vi "GetDataForExcel.ExtractData.vi"(7 "Report Type":i32, 8 "Error In":errorcluster, 10 "Folders":string[](array[string]), 11 "Path":path) -> (0 "Error Out":errorcluster, 2 "Data":dbl[][](array[numeric]), 3 "Names":string[](array[string]))   [LabVIEW 2013, in "main.lvlib"]
uses:
  main.lvlib
  Controls/Enum Variables.ctl
  <userlib>/_MGI/Error Handling/MGI Suppress Error Code/MGI Suppress Error Code (Scalar).vi
  <userlib>/_OpenG.lib/file/file.llb/File Exists - Scalar__ogtk.vi
  <vilib>/Utility/file.llb/Read From Spreadsheet File (string).vi
  <vilib>/Utility/file.llb/Read From Spreadsheet File (DBL).vi
  <vilib>/regexp/Match Regular Expression.xnode
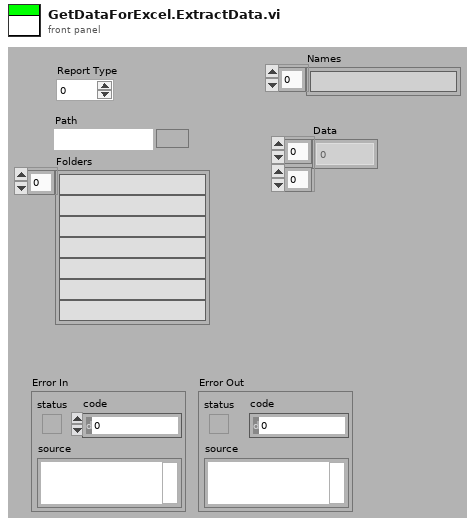
[diagram p1: front panel]
types:
  T1 = typedef "main.lvlib/Enum Variables.ctl" = enum16{"SetAcqFilter", "GetAcqFilter", "Set Filter", "Get Filter", "Set Height", "Get Height", "Set Recorded Height", "Get Recorded Height", "Set Blue Pressure", "Get Blue Pressure", "Set Red Pressure", "Get Red Pressure", "Init", "Reset Pressure", "Set Red Cursors", "Get Red Cursors", "Set Blue Cursors", "Get Blue Cursors", "Set Language", "Get Language", "Set Active Graphs", "Get ActiveGraphs", "Set Method", "Get Method", "Set Encryption", "Get Encryption", "Set ExcelVersion", "Get ExcelVersion", "Set DICOM Avail", "Get DICOM Avail", "Set DICOM Encode", "Get DICOM Encode", "Set JournalExport", "Get JournalExport", "Set Sequence", "Get Sequence", "Set DAQ Connected", "Get DAQ Connected", "Set Current Graph", "Get Current Graph", "Set General Settings", "Get Hyphenation", "Set Arm Calc Method", "Get Arm Calc Method", "Set Dicom Tags", "Get Dicom Tags", "Set BT Serial", "Get BT Serial", "Set BT Accepted Serials", "Get BT Accepted Serials", "Get BT License", "Set BT License"}
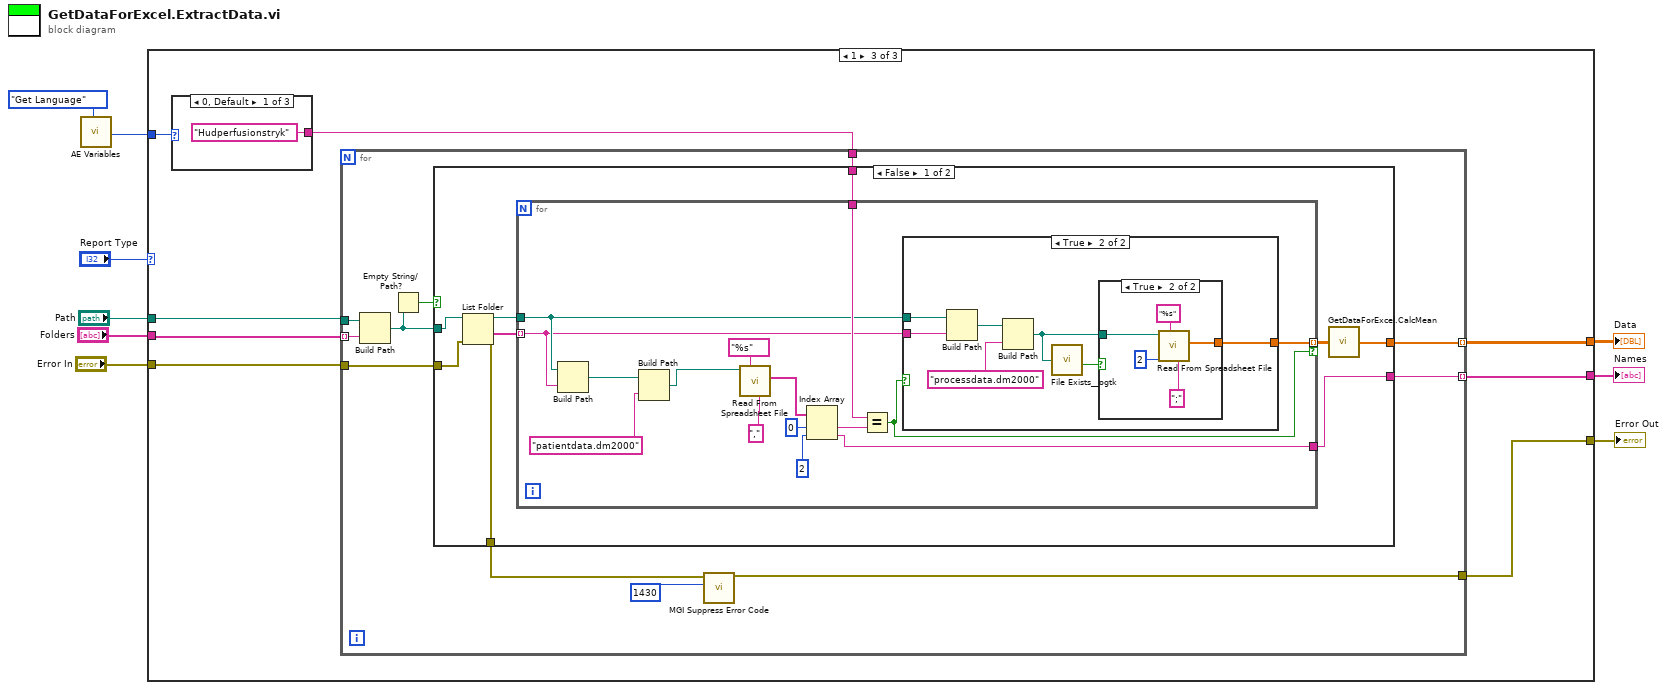
[diagram p0: block diagram]
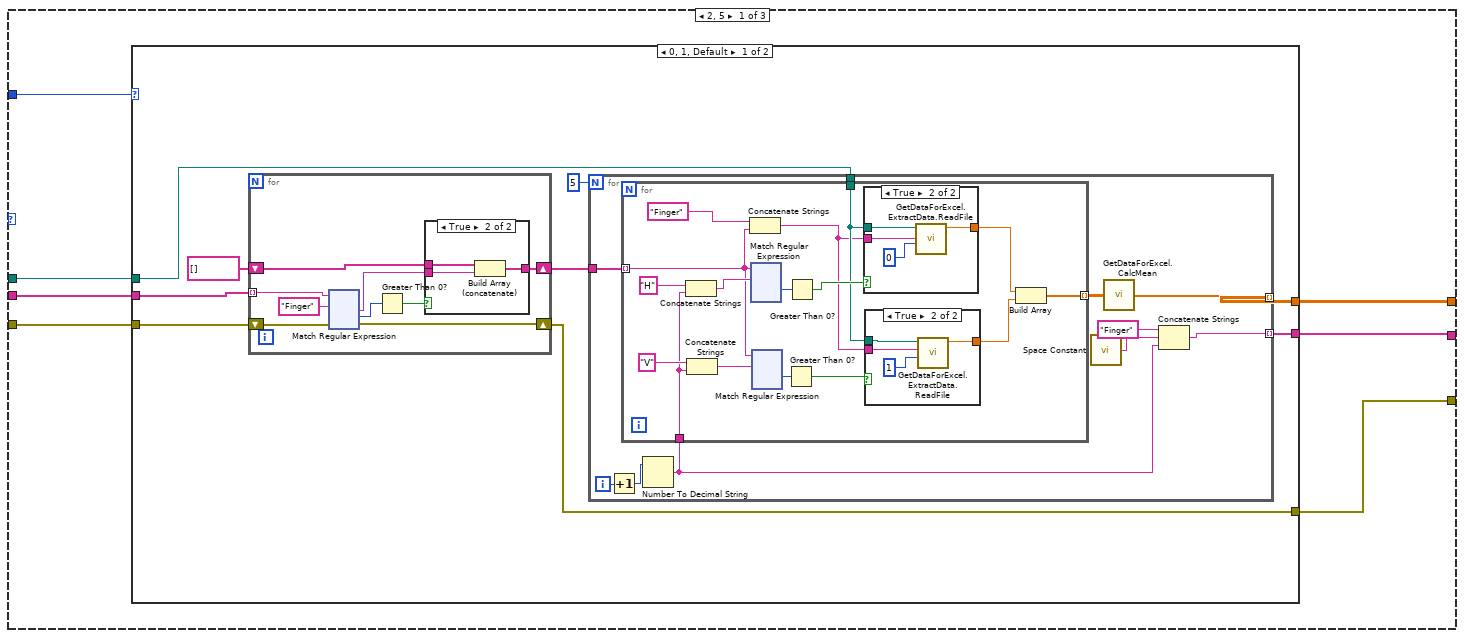
[diagram p2: hidden frame]
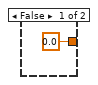
[diagram p3: hidden frame]
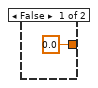
[diagram p4: hidden frame]
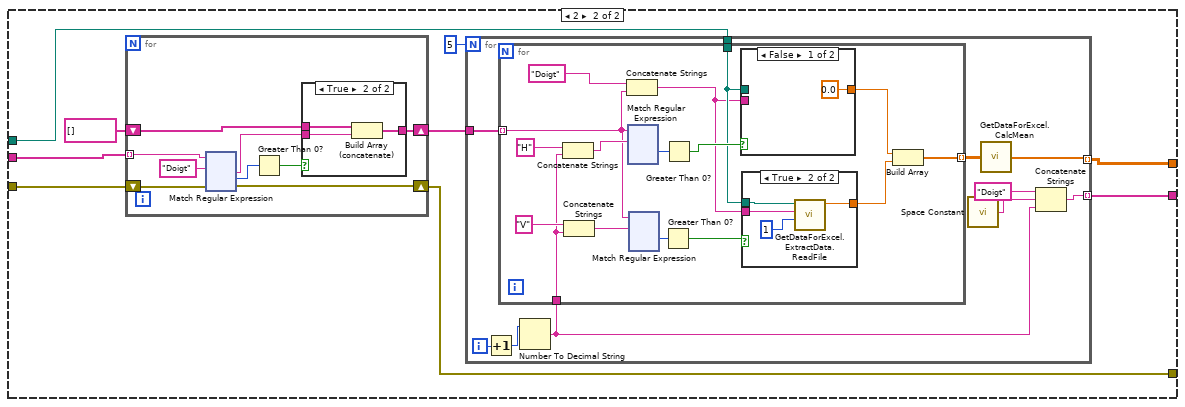
[diagram p6: hidden frame]
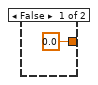
[diagram p7: hidden frame]
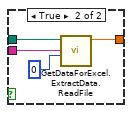
[diagram p8: hidden frame]
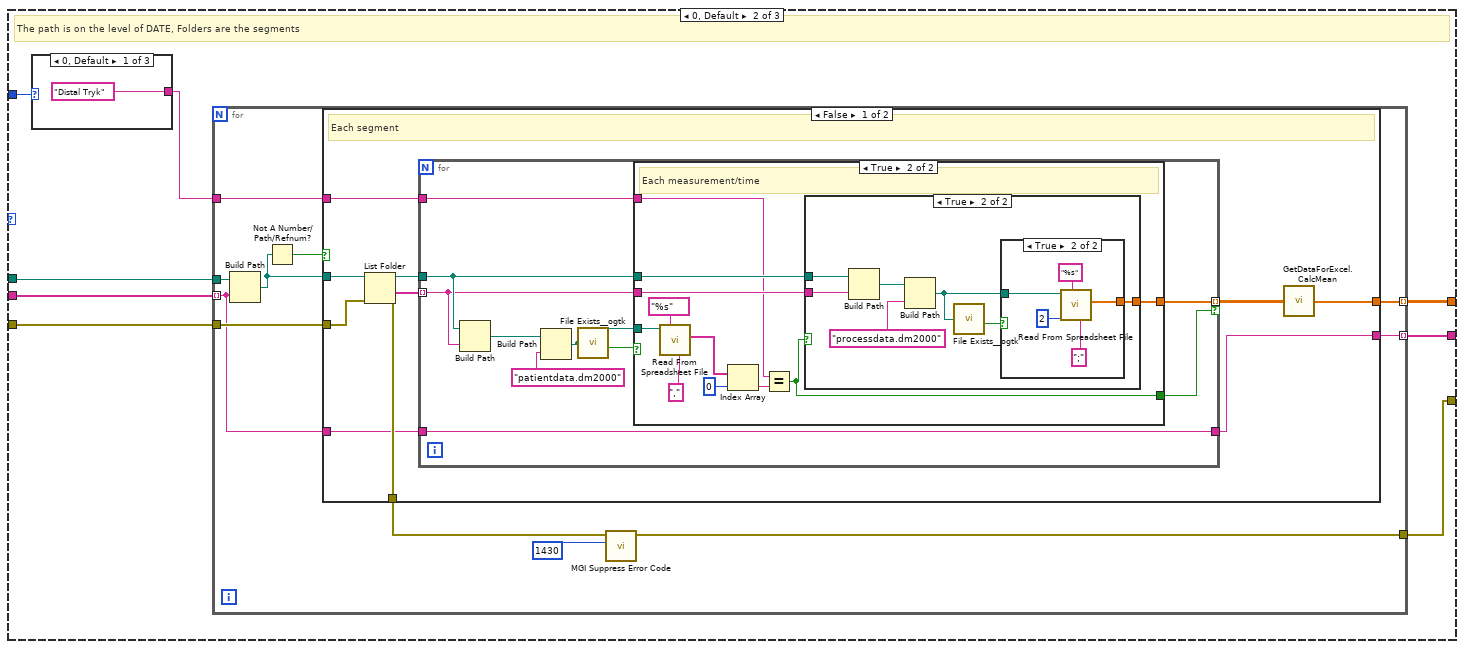
[diagram p10: hidden frame]
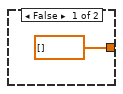
[diagram p13: hidden frame]
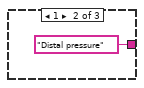
[diagram p15: hidden frame]
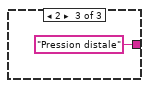
[diagram p16: hidden frame]
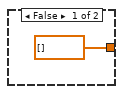
[diagram p18: hidden frame]
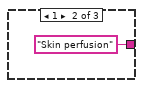
[diagram p20: hidden frame]
diagram:
  n1 = call "AE Variables.vi"("Action"=Enum_Variables."Get Language") -> ("RingOut"=w1:u16)  [unwired: 11 in, 7 out]
  n2 = case shown="1" "Report Type" {
    tunnel: [w15 w800 w866] -> w9
    tunnel: "Folders" -> [w14 w801 w871]
    tunnel: "Path" -> [w13 w802 w872]
    tunnel: "Error In" -> [w16 w803 w870]
    tunnel: [w12 w805 w868] -> w5
    tunnel: [w11 w804 w867] -> w4
    tunnel: w1 -> [w10 w806 w873]
    frame 2, 5 {
      n3 = case shown="0, 1, Default" w10 {
        tunnel: w16 -> [w25 w416]
        tunnel: [w24 w415] -> w15
        tunnel: w14 -> [w23 w414]
        tunnel: w13 -> [w20 w411]
        tunnel: [w19 w410] -> w12
        tunnel: [w18 w409] -> w11
        frame 0, 1, Default {
          n4 = for {
            shift-right: [w290] -> w24
            shift-left: w25 -> [w291]
            shift-right: [w289] -> w22
            shift-left: string[] [] -> [w288]
            tunnel: w23 -> [w285] mode=indexing
            n5 = xnode "Match Regular Expression"("input string"=w285, "regular expression"="Finger", "error in"=w291) -> ("after match"=w284:string, "offset past match"=w286:i32, "error out"=w290:errorcluster)  [unwired: 3 in, 2 out]
            n6 = Greater Than 0?(x=w286) -> (x > 0?=w287:bool)
            n7 = case shown="True" w287 {
              tunnel: [w293 w296] -> w289
              tunnel: w288 -> [w293 w295]
              tunnel: w284 -> [_ w294]
              frame False {
              }
              frame True {
                n8 = Build Array (concatenate)(w295, w294) -> (w296:string[])
              }
            }
          }
          n9 = for {
            N: 5 -> [_]
            tunnel: w22 -> [w35]
            tunnel: w20 -> [w32]
            tunnel: [w30] -> w19 mode=indexing
            tunnel: [w29] -> w18 mode=indexing
            i -> [w34]
            n10 = Increment(x=w34) -> (x+1=w33:i32)
            n11 = Number To Decimal String(number=w33) -> (decimal integer string=w26:string)  [unwired: 1 in]
            n12 = for {
              tunnel: w35 -> [w36] mode=indexing
              tunnel: w26 -> [w48]
              tunnel: w32 -> [w41]
              tunnel: [w38] -> w31 mode=indexing
              n13 = Concatenate Strings("H", w48) -> (w47:string)
              n14 = Concatenate Strings("V", w48) -> (w49:string)
              n15 = Concatenate Strings("Finger" ("string"), w36) -> (w37:string)
              n16 = xnode "Match Regular Expression"("input string"=w36, "regular expression"=w47) -> ("offset past match"=w46:i32)  [unwired: 4 in, 4 out]
              n17 = xnode "Match Regular Expression"("input string"=w36, "regular expression"=w49) -> ("offset past match"=w45:i32)  [unwired: 4 in, 4 out]
              n18 = Greater Than 0?(x=w45) -> (x > 0?=w42:bool)
              n19 = Greater Than 0?(x=w46) -> (x > 0?=w44:bool)
              n20 = case shown="True" w44 {
                tunnel: w41 -> [_ w61]
                tunnel: w37 -> [_ w60]
                tunnel: [0.0 ("data") w59] -> w40
                frame False {
                }
                frame True {
                  n21 = call "GetDataForExcel.ExtractData.ReadFile.vi"("index"=0, "relative path"=w60, "base path"=w61) -> ("data"=w59:dbl)  [unwired: 8 in]
                }
              }
              n22 = case shown="True" w42 {
                tunnel: w37 -> [_ w56]
                tunnel: w41 -> [_ w55]
                tunnel: [0.0 ("data") w54] -> w39
                frame False {
                }
                frame True {
                  n23 = call "GetDataForExcel.ExtractData.ReadFile.vi"("index"=1, "relative path"=w56, "base path"=w55) -> ("data"=w54:dbl)  [unwired: 8 in]
                }
              }
              n24 = Build Array(w40, w39) -> (w38:dbl[])
            }
            n25 = call <vilib>:"Space Constant.vi"() -> ("String"=w27:string)
            n26 = call "GetDataForExcel.CalcMean.vi"("Input Array"=w31) -> ("Array"=w30:dbl[])
            n27 = Concatenate Strings("Finger", w27, w26) -> (w29:string)
          }
        }
        frame 2 {
          n28 = for {
            shift-right: [w681] -> w415
            shift-left: w416 -> [w682]
            shift-right: [w680] -> w413
            shift-left: string[] [] -> [w679]
            tunnel: w414 -> [w676] mode=indexing
            n29 = xnode "Match Regular Expression"("input string"=w676, "regular expression"="Doigt", "error in"=w682) -> ("after match"=w675:string, "offset past match"=w677:i32, "error out"=w681:errorcluster)  [unwired: 3 in, 2 out]
            n30 = Greater Than 0?(x=w677) -> (x > 0?=w678:bool)
            n31 = case shown="True" w678 {
              tunnel: [w684 w687] -> w680
              tunnel: w679 -> [w684 w686]
              tunnel: w675 -> [_ w685]
              frame False {
              }
              frame True {
                n32 = Build Array (concatenate)(w686, w685) -> (w687:string[])
              }
            }
          }
          n33 = for {
            N: 5 -> [_]
            tunnel: w413 -> [w426]
            tunnel: w411 -> [w423]
            tunnel: [w421] -> w410 mode=indexing
            tunnel: [w420] -> w409 mode=indexing
            i -> [w425]
            n34 = Increment(x=w425) -> (x+1=w424:i32)
            n35 = Number To Decimal String(number=w424) -> (decimal integer string=w417:string)  [unwired: 1 in]
            n36 = for {
              tunnel: w426 -> [w427] mode=indexing
              tunnel: w417 -> [w439]
              tunnel: w423 -> [w432]
              tunnel: [w429] -> w422 mode=indexing
              n37 = Concatenate Strings("H", w439) -> (w438:string)
              n38 = Concatenate Strings("V", w439) -> (w440:string)
              n39 = Concatenate Strings("Doigt" ("string"), w427) -> (w428:string)
              n40 = xnode "Match Regular Expression"("input string"=w427, "regular expression"=w438) -> ("offset past match"=w437:i32)  [unwired: 4 in, 4 out]
              n41 = xnode "Match Regular Expression"("input string"=w427, "regular expression"=w440) -> ("offset past match"=w436:i32)  [unwired: 4 in, 4 out]
              n42 = Greater Than 0?(x=w436) -> (x > 0?=w433:bool)
              n43 = Greater Than 0?(x=w437) -> (x > 0?=w435:bool)
              n44 = case shown="False" w435 {
                tunnel: w432 -> [_ w452]
                tunnel: w428 -> [_ w451]
                tunnel: [0.0 ("data") w450] -> w431
                frame False {
                }
                frame True {
                  n45 = call "GetDataForExcel.ExtractData.ReadFile.vi"("index"=0, "relative path"=w451, "base path"=w452) -> ("data"=w450:dbl)  [unwired: 8 in]
                }
              }
              n46 = case shown="True" w433 {
                tunnel: w428 -> [_ w447]
                tunnel: w432 -> [_ w446]
                tunnel: [0.0 ("data") w445] -> w430
                frame False {
                }
                frame True {
                  n47 = call "GetDataForExcel.ExtractData.ReadFile.vi"("index"=1, "relative path"=w447, "base path"=w446) -> ("data"=w445:dbl)  [unwired: 8 in]
                }
              }
              n48 = Build Array(w431, w430) -> (w429:dbl[])
            }
            n49 = call <vilib>:"Space Constant.vi"() -> ("String"=w418:string)
            n50 = call "GetDataForExcel.CalcMean.vi"("Input Array"=w422) -> ("Array"=w421:dbl[])
            n51 = Concatenate Strings("Doigt", w418, w417) -> (w420:string)
          }
        }
      }
    }
    frame 0, Default {
      # "The path is on the level of DATE, Folders are the segments"
      n52 = case shown="0, Default" w806 {
        tunnel: ["Distal Tryk" "Distal pressure" "Pression distale"] -> w799
        frame 0, Default {
        }
        frame 1 {
        }
        frame 2 {
        }
      }
      n53 = for {
        tunnel: [w815] -> w800
        tunnel: [w817] -> w805 mode=indexing
        tunnel: [w813] -> w804 mode=indexing
        tunnel: w803 -> [w812]
        tunnel: w802 -> [w811]
        tunnel: w801 -> [w807] mode=indexing
        tunnel: w799 -> [w808]
        n54 = Build Path(base path=w811, name or relative path=w807) -> (appended path=w810:path)
        n55 = Not A Number/Path/Refnum?(number/path/refnum=w810) -> (NaN/Path/Refnum?=w809:bool)
        n56 = case shown="False" w809 {
          tunnel: [w824 _] -> w817
          tunnel: [w823 w862] -> w816
          tunnel: [w822 _] -> w813
          tunnel: w812 -> [w821 w862]
          tunnel: w810 -> [w820 _]
          tunnel: w808 -> [w819 _]
          tunnel: w807 -> [w818 _]
          frame False {
            # "Each segment"
            n57 = List Folder(path=w820, error in=w821) -> (path out=w827:path, folder names=w825:string[], error out=w823:errorcluster)  [unwired: 2 in, 1 out]
            n58 = for {
              tunnel: w825 -> [w829] mode=indexing
              tunnel: w827 -> [w835]
              tunnel: [w837] -> w826 mode=indexing if=w836
              tunnel: [w828] -> w822
              tunnel: w819 -> [w830]
              tunnel: w818 -> [w828]
              n59 = Build Path(base path=w835, name or relative path=w829) -> (appended path=w834:path)
              n60 = Build Path(base path=w834, name or relative path="patientdata.dm2000") -> (appended path=w832:path)
              n61 = call-poly <userlib>:"File Exists__ogtk.vi"("file path"=w832) -> ("exists"=w831:bool)  [unwired: 6 in, 1 out]
              n62 = case shown="True" w831 {
                tunnel: [_ w848] -> w837
                tunnel: [_ w843] -> w836
                tunnel: w835 -> [_ w841]
                tunnel: w829 -> [_ w840]
                tunnel: w832 -> [_ w839]
                tunnel: w830 -> [_ w838]
                frame False {
                }
                frame True {
                  # "Each measurement/time"
                  n63 = call-poly <vilib>:"Read From Spreadsheet File.vi"("delimiter (\\t)"="," ("delimiter (\\t)"), "format (%s)"="%s", "file path (dialog if empty)"=w839) -> ("first row"=w844:string[])  [unwired: 4 in, 4 out]
                  n64 = Index Array(array=w844, index=0 ("index (row)")) -> (element=w842:string)
                  n65 = Equal?(x=w838, y=w842) -> (x = y?=w843:bool)
                  n66 = case shown="True" w843 {
                    tunnel: w841 -> [_ w855]
                    tunnel: w840 -> [_ w854]
                    tunnel: [_ w853] -> w848
                    frame False {
                    }
                    frame True {
                      n67 = Build Path(base path=w855, name or relative path=w854) -> (appended path=w851:path)
                      n68 = Build Path(base path=w851, name or relative path="processdata.dm2000") -> (appended path=w849:path)
                      n69 = call-poly <userlib>:"File Exists__ogtk.vi"("file path"=w849) -> ("exists"=w850:bool)  [unwired: 6 in, 1 out]
                      n70 = case shown="True" w850 {
                        tunnel: [dbl[] [] w859] -> w853
                        tunnel: w849 -> [_ w857]
                        frame False {
                        }
                        frame True {
                          n71 = call-poly <vilib>:"Read From Spreadsheet File.vi"("delimiter (\\t)"=";" ("delimiter (\\t)"), "format (%.3f)"="%s", "max characters/row  (no limit:0)"=2, "file path (dialog if empty)"=w857) -> ("first row"=w859:dbl[])  [unwired: 3 in, 4 out]
                        }
                      }
                    }
                  }
                }
              }
            }
            n72 = call "GetDataForExcel.CalcMean.vi"("Input Array"=w826) -> ("Array"=w824:dbl[])
          }
          frame True {
          }
        }
        n73 = call-poly <userlib>:"MGI Suppress Error Code.vi"("Error Code"=1430, "Error In"=w816) -> ("Error Out"=w815:errorcluster)  [unwired: 4 in, 1 out]
      }
    }
    frame 1 {
      n74 = case shown="0, Default" w873 {
        tunnel: ["Hudperfusionstryk" "Skin perfusion" "Perfusion cutanée"] -> w869
        frame 0, Default {
        }
        frame 1 {
        }
        frame 2 {
        }
      }
      n75 = for {
        tunnel: [w882] -> w866
        tunnel: [w884] -> w868 mode=indexing
        tunnel: [w880] -> w867 mode=indexing
        tunnel: w870 -> [w879]
        tunnel: w869 -> [w878]
        tunnel: w872 -> [w877]
        tunnel: w871 -> [w876] mode=indexing
        n76 = Build Path(base path=w877, name or relative path=w876) -> (appended path=w875:path)
        n77 = Empty String/Path?(string/path=w875) -> (empty?=w874:bool)
        n78 = case shown="False" w874 {
          tunnel: w875 -> [w893 _]
          tunnel: [w889 _] -> w884
          tunnel: [w888 w922] -> w883
          tunnel: [w887 _] -> w880
          tunnel: w879 -> [w886 w922]
          tunnel: w878 -> [w885 _]
          frame False {
            n79 = List Folder(path=w893, error in=w886) -> (path out=w892:path, folder names=w890:string[], error out=w888:errorcluster)  [unwired: 2 in, 1 out]
            n80 = for {
              tunnel: w890 -> [w897] mode=indexing
              tunnel: w892 -> [w898]
              tunnel: [w908] -> w891 mode=indexing if=w903
              tunnel: [w900] -> w887
              tunnel: w885 -> [w899]
              n81 = Build Path(base path=w898, name or relative path=w897) -> (appended path=w896:path)
              n82 = Build Path(base path=w896, name or relative path="patientdata.dm2000") -> (appended path=w894:path)
              n83 = call-poly <vilib>:"Read From Spreadsheet File.vi"("delimiter (\\t)"="," ("delimiter (\\t)"), "format (%s)"="%s", "file path (dialog if empty)"=w894) -> ("first row"=w904:string[])  [unwired: 4 in, 4 out]
              n84 = Index Array(array=w904, index #1=0 ("index (row)"), index #2=2 ("index")) -> (element #1=w902:string, element #2=w900:string)
              n85 = Equal?(x=w899, y=w902) -> (x = y?=w903:bool)
              n86 = case shown="True" w903 {
                tunnel: w898 -> [_ w915]
                tunnel: w897 -> [_ w914]
                tunnel: [_ w913] -> w908
                frame False {
                }
                frame True {
                  n87 = Build Path(base path=w915, name or relative path=w914) -> (appended path=w911:path)
                  n88 = Build Path(base path=w911, name or relative path="processdata.dm2000") -> (appended path=w909:path)
                  n89 = call-poly <userlib>:"File Exists__ogtk.vi"("file path"=w909) -> ("exists"=w910:bool)  [unwired: 6 in, 1 out]
                  n90 = case shown="True" w910 {
                    tunnel: [dbl[] [] w919] -> w913
                    tunnel: w909 -> [_ w917]
                    frame False {
                    }
                    frame True {
                      n91 = call-poly <vilib>:"Read From Spreadsheet File.vi"("delimiter (\\t)"=";" ("delimiter (\\t)"), "format (%.3f)"="%s", "max characters/row  (no limit:0)"=2, "file path (dialog if empty)"=w917) -> ("first row"=w919:dbl[])  [unwired: 3 in, 4 out]
                    }
                  }
                }
              }
            }
            n92 = call "GetDataForExcel.CalcMean.vi"("Input Array"=w891) -> ("Array"=w889:dbl[])
          }
          frame True {
          }
        }
        n93 = call-poly <userlib>:"MGI Suppress Error Code.vi"("Error Code"=1430, "Error In"=w883) -> ("Error Out"=w882:errorcluster)  [unwired: 4 in, 1 out]
      }
    }
  }
  "Error Out" <- w9
  "Data" <- w5
  "Names" <- w4
